vi "Alicat error reconnect.vi"(8 "error in (no error)":errorcluster, 11 "AlicatPressureController in":refnum<class "AlicatPressureController.lvclass">) -> (0 "error out":errorcluster, 3 "AlicatPressureController out":refnum<class "AlicatPressureController.lvclass">)   [LabVIEW 2020, in "AlicatPressureController.lvclass"]
uses:
  AlicatPressureController.lvclass
  AlicatPressureController.lvclass/AlicatPressureController.ctl
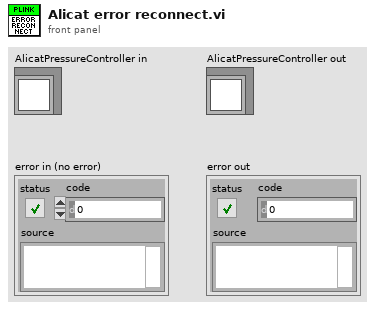
[diagram p1: front panel]
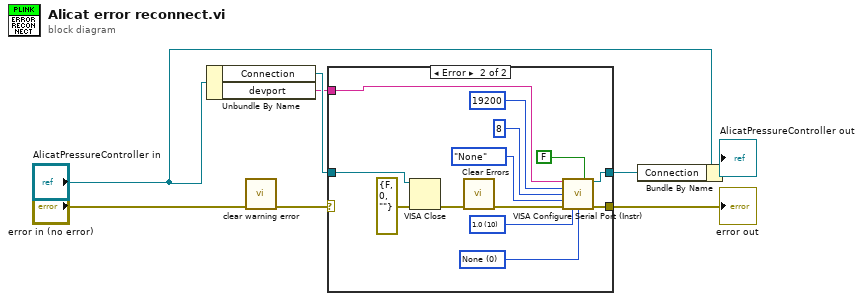
[diagram p0: block diagram]
diagram:
  n1 = Unbundle By Name("AlicatPressureController in") -> ("Connection"=w5:refnum<visa-resource-name>, "devport"=w4:string)
  n2 = call "clear warning error.vi"("error in"="error in (no error)") -> ("error out"=w2:errorcluster)  [unwired: 10 in]
  n3 = case shown="Error" w2 {
    selector: w2 -> [w10 _]
    tunnel: [w9 w16] -> w3
    tunnel: [w10 w15] -> w8
    tunnel: w5 -> [w9 w11]
    tunnel: w4 -> [_ w12]
    frame No Error {
    }
    frame Error {
      w22 = u16 0 items=["None", "XON/XOFF", "RTS/CTS", "XON/XOFF & RTS/CTS", "DTR/DSR", "XON/XOFF & DTR/DSR"] ("flow control (0:none)")
      w21 = u16 10 items=["1.0"=10, "1.5"=15, "2.0"=20] ("stop bits (10: 1 bit)")
      n4 = VISA Close(VISA resource name=w11, error in (no error)=errorcluster {"status"=FALSE, "code"=0, "source"=""}) -> (error out=w14:errorcluster)
      n5 = call "Clear Errors.vi"("error in (no error)"=w14) -> ("error out"=w13:errorcluster)  [unwired: 5 in, 1 out]
      n6 = call "VISA Configure Serial Port (Instr).vi"("VISA resource name"=w12, "Enable Termination\nChar (T)"=FALSE ("Enable Termination\nChar (T)"), "baud rate (9600)"=u32 19200, "data bits (8)"=u16 8, "parity (0:none)"=enum16{"None", "Odd", "Even", "Mark", "Space"}."None", "error in (no error)"=w13, "stop bits (10: 1 bit)"=w21, "flow control (0:none)"=w22) -> ("VISA resource name out"=w16:refnum<visa-resource-name>, "error out"=w15:errorcluster)  [unwired: 6 in]
    }
  }
  "error out" <- w8
  n7 = Bundle By Name(cluster="AlicatPressureController in", "Connection"=w3) -> (→"AlicatPressureController out":refnum<class "AlicatPressureController.lvclass">)
